vi "7. 绘制：管道内的 数据点分布 图.vi"(0 ">1000 数据点 红色":u32(colorbox)=13107200, 3 "<120 数据点 灰色":u32(colorbox)=11121611, 4 "<1000 数据点 橘色":u32(colorbox)=16732970, 5 "<-120 数据点 青色":u32(colorbox)=2817023, 6 "<400 数据点 黄色":u32(colorbox)=16769858, 7 "<-300 数据点 蓝色":u32(colorbox)=16777224, 8 "管道分布":picture, 9 "输入：放大倍数":i32, 10 "光纤分布":dbl[][](array[numeric]), 11 "数据分布 一维数组":dbl[](array[numeric]) format="%#_13g") -> (2 "管道+数据分布":picture)   [LabVIEW 2018]
panel:
  in  "fill?(F)":bool caption="填充？(F)"
  in  ">1000 数据点 画笔":T1={"Width"=8, "Style"=enum."Solid"}
  in  "<1000 数据点 画笔":T1={"Width"=8, "Style"=enum."Solid"}
  in  "<400 数据点 画笔":T1={"Width"=8, "Style"=enum."Solid"}
  in  ">1000 数据点：光纤+数据 分布":cluster{"x":dbl, "y":dbl, "数据":dbl, "索引":i32}[](array[cluster])
  in  "<1000 数据点：光纤+数据 分布":cluster{"x":dbl, "y":dbl, "数据":dbl, "索引":i32}[](array[cluster])
  in  "<400 数据点：光纤+数据 分布":cluster{"x":dbl, "y":dbl, "数据":dbl, "索引":i32}[](array[cluster])
  in  "<120 数据点 画笔":T1={"Width"=8, "Style"=enum."Solid"}
  in  "<-120 数据点 画笔":T1={"Width"=8, "Style"=enum."Solid"}
  in  "<120 数据点：光纤+数据 分布":cluster{"x":dbl, "y":dbl, "数据":dbl, "索引":i32}[](array[cluster])
  in  "<-120 数据点：光纤+数据 分布":cluster{"x":dbl, "y":dbl, "数据":dbl, "索引":i32}[](array[cluster])
  in  "<-300 数据点：光纤+数据 分布":cluster{"x":dbl, "y":dbl, "数据":dbl, "索引":i32}[](array[cluster])
  in  "<-300 数据点 画笔":T1={"Width"=8, "Style"=enum."Solid"}
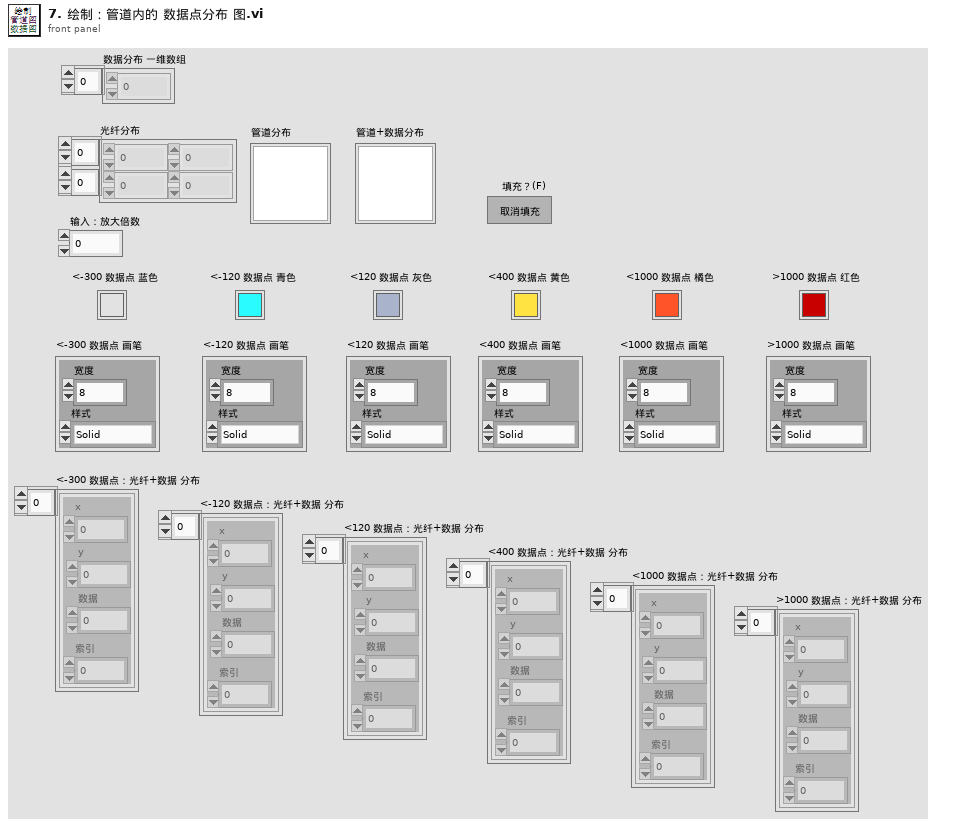
[diagram p1: front panel]
types:
  T1 = cluster{"Width":u16, "Style":enum32{"Solid", "Dash", "Dot", "DashDot", "DashDotDot"}}
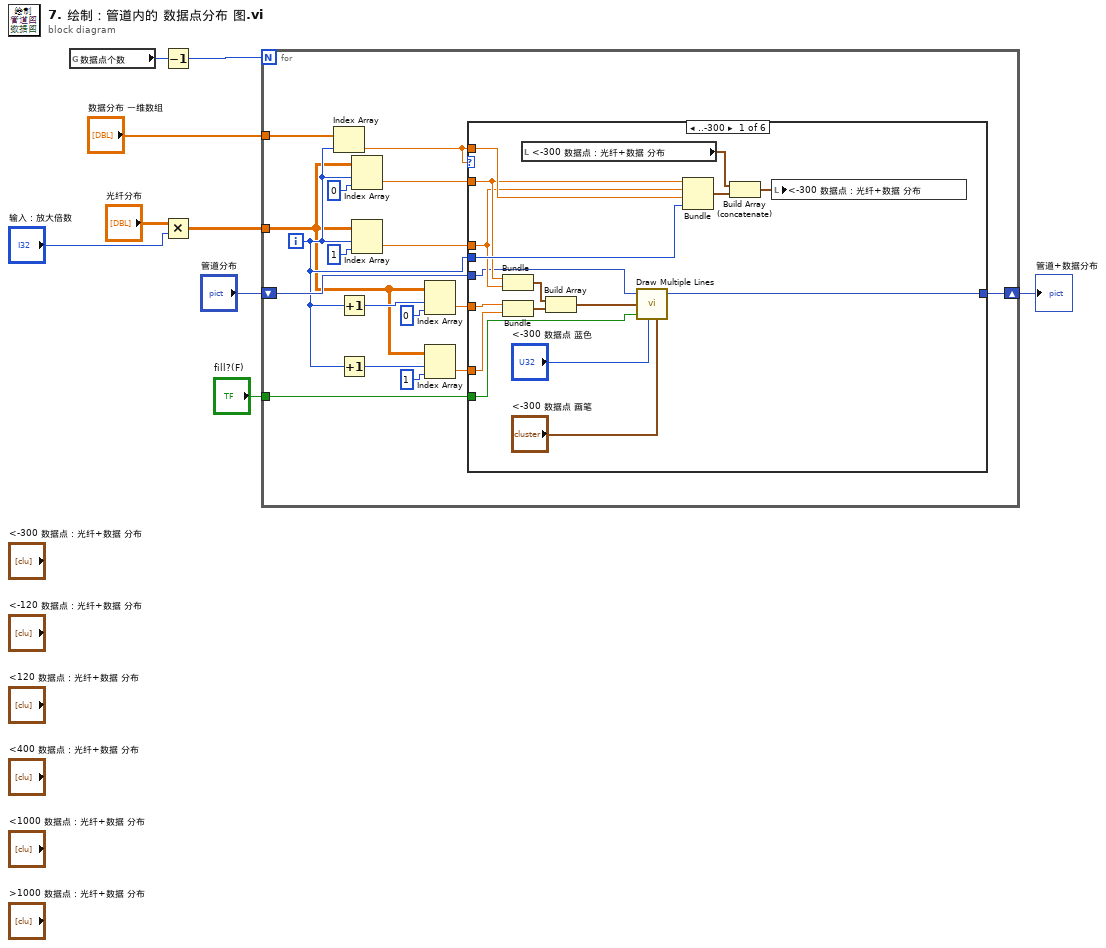
[diagram p0: block diagram]
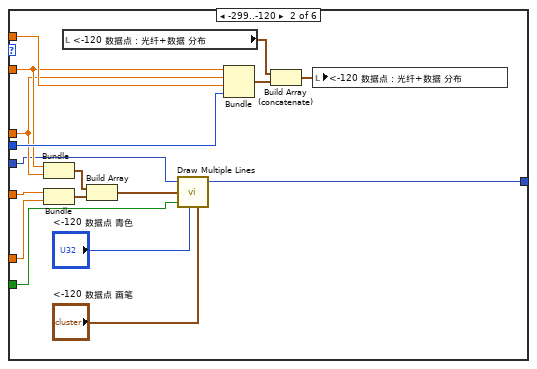
[diagram p2: hidden frame]
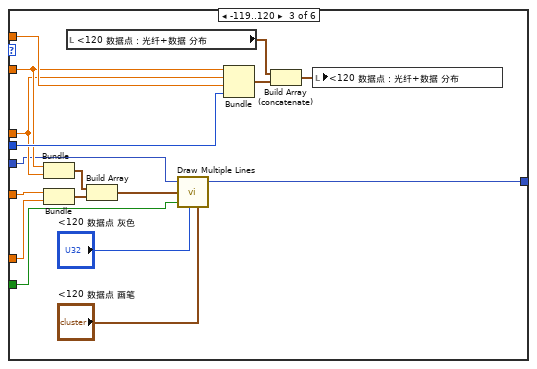
[diagram p3: hidden frame]
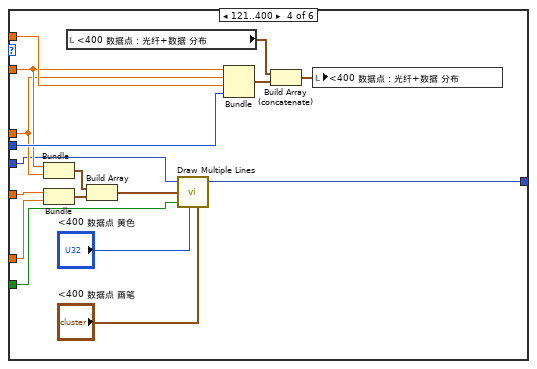
[diagram p4: hidden frame]
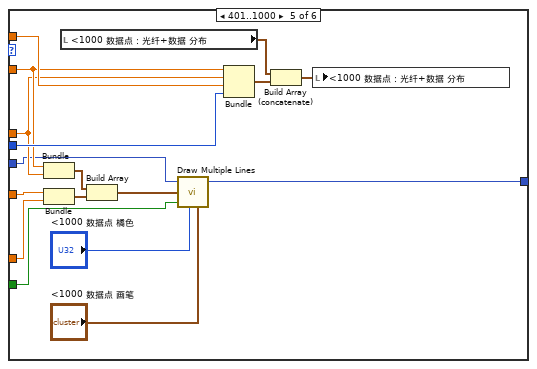
[diagram p5: hidden frame]
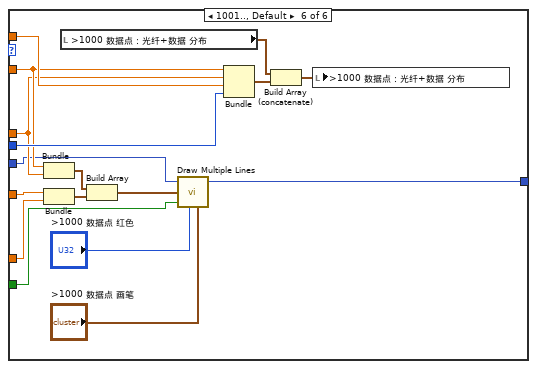
[diagram p6: hidden frame]
diagram:
  n1 = global read "全局变量：数据点个数.vi" "数据点个数"() -> (w2:i32)
  n2 = Decrement(x=w2) -> (x-1=w1:i32)
  n3 = Multiply(x="光纤分布", y="输入：放大倍数") -> (x*y=w9:dbl[][])
  n4 = for {
    N: w1 -> [_]
    tunnel: "数据分布 一维数组" -> [w26]
    tunnel: w9 -> [w13]
    shift-right: [w23] -> w4
    shift-left: "管道分布" -> [w20]
    tunnel: "fill?(F)" -> [w10]
    i -> [w14]
    n5 = Index Array(array=w26, index=w14) -> (element=w19:dbl)
    n6 = Increment(x=w14) -> (x+1=w16:i32)
    n7 = Increment(x=w14) -> (x+1=w15:i32)
    n8 = Index Array(array=w13, index (row)=w14, index (col)=0) -> (element=w22:dbl)
    n9 = Index Array(array=w13, index (row)=w14, index (col)=1) -> (element=w21:dbl)
    n10 = Index Array(array=w13, index (row)=w16, index (col)=0) -> (element=w12:dbl)
    n11 = Index Array(array=w13, index (row)=w15, index (col)=1) -> (element=w11:dbl)
    n12 = case shown="..-300" w19 {
      tunnel: w14 -> [w43 w60 w77 w94 w111 w128]
      tunnel: w19 -> [w42 w59 w76 w93 w110 w127]
      tunnel: w22 -> [w41 w58 w75 w92 w109 w126]
      tunnel: w21 -> [w40 w57 w74 w91 w108 w125]
      tunnel: w20 -> [w29 w47 w64 w79 w95 w113]
      tunnel: [w28 w48 w65 w82 w99 w112] -> w23
      tunnel: w12 -> [w36 w53 w70 w87 w104 w121]
      tunnel: w11 -> [w35 w52 w69 w86 w103 w120]
      tunnel: w10 -> [w27 w44 w61 w78 w98 w119]
      frame ..-300 {
        n13 = Bundle(w41, w40) -> (w33:cluster{dbl, dbl})  [unwired: 1 in]
        n14 = Bundle(w36, w35) -> (w34:cluster{dbl, dbl})  [unwired: 1 in]
        n15 = local read "<-300 数据点：光纤+数据 分布"() -> (w37:cluster{"x":dbl, "y":dbl, "数据":dbl, "索引":i32}[])
        n16 = Build Array(w33, w34) -> (w32:cluster{dbl, dbl}[])
        n17 = call <vilib>:"Draw Multiple Lines.vi"("picture"=w29, "line endpoints"=w32, "fill?(F)"=w27, "color(black)"="<-300 数据点 蓝色", "pen"="<-300 数据点 画笔") -> ("new picture"=w28:picture)  [unwired: 4 in]
        n18 = Bundle(w41, w40, "数值"=w42, w43) -> (w39:cluster{dbl, dbl, "数值":dbl, i32})  [unwired: 1 in]
        n19 = Build Array (concatenate)(w37, w39) -> (w38:cluster{"x":dbl, "y":dbl, "数值":dbl, "索引":i32}[])
        n20 = local write "<-300 数据点：光纤+数据 分布"(w38) -> ()
      }
      frame -299..-120 {
        n21 = Bundle(w58, w57) -> (w50:cluster{dbl, dbl})  [unwired: 1 in]
        n22 = Bundle(w53, w52) -> (w51:cluster{dbl, dbl})  [unwired: 1 in]
        n23 = local read "<-120 数据点：光纤+数据 分布"() -> (w54:cluster{"x":dbl, "y":dbl, "数据":dbl, "索引":i32}[])
        n24 = Build Array(w50, w51) -> (w49:cluster{dbl, dbl}[])
        n25 = call <vilib>:"Draw Multiple Lines.vi"("picture"=w47, "line endpoints"=w49, "fill?(F)"=w44, "color(black)"="<-120 数据点 青色", "pen"="<-120 数据点 画笔") -> ("new picture"=w48:picture)  [unwired: 4 in]
        n26 = Bundle(w58, w57, "数值"=w59, w60) -> (w56:cluster{dbl, dbl, "数值":dbl, i32})  [unwired: 1 in]
        n27 = Build Array (concatenate)(w54, w56) -> (w55:cluster{"x":dbl, "y":dbl, "数值":dbl, "索引":i32}[])
        n28 = local write "<-120 数据点：光纤+数据 分布"(w55) -> ()
      }
      frame -119..120 {
        n29 = Bundle(w75, w74) -> (w67:cluster{dbl, dbl})  [unwired: 1 in]
        n30 = Bundle(w70, w69) -> (w68:cluster{dbl, dbl})  [unwired: 1 in]
        n31 = local read "<120 数据点：光纤+数据 分布"() -> (w71:cluster{"x":dbl, "y":dbl, "数据":dbl, "索引":i32}[])
        n32 = Build Array(w67, w68) -> (w66:cluster{dbl, dbl}[])
        n33 = call <vilib>:"Draw Multiple Lines.vi"("picture"=w64, "line endpoints"=w66, "fill?(F)"=w61, "color(black)"="<120 数据点 灰色", "pen"="<120 数据点 画笔") -> ("new picture"=w65:picture)  [unwired: 4 in]
        n34 = Bundle(w75, w74, "数值"=w76, w77) -> (w73:cluster{dbl, dbl, "数值":dbl, i32})  [unwired: 1 in]
        n35 = Build Array (concatenate)(w71, w73) -> (w72:cluster{"x":dbl, "y":dbl, "数值":dbl, "索引":i32}[])
        n36 = local write "<120 数据点：光纤+数据 分布"(w72) -> ()
      }
      frame 121..400 {
        n37 = Bundle(w92, w91) -> (w84:cluster{dbl, dbl})  [unwired: 1 in]
        n38 = Bundle(w87, w86) -> (w85:cluster{dbl, dbl})  [unwired: 1 in]
        n39 = local read "<400 数据点：光纤+数据 分布"() -> (w88:cluster{"x":dbl, "y":dbl, "数据":dbl, "索引":i32}[])
        n40 = Build Array(w84, w85) -> (w83:cluster{dbl, dbl}[])
        n41 = call <vilib>:"Draw Multiple Lines.vi"("picture"=w79, "line endpoints"=w83, "fill?(F)"=w78, "color(black)"="<400 数据点 黄色", "pen"="<400 数据点 画笔") -> ("new picture"=w82:picture)  [unwired: 4 in]
        n42 = Bundle(w92, w91, "数值"=w93, w94) -> (w90:cluster{dbl, dbl, "数值":dbl, i32})  [unwired: 1 in]
        n43 = Build Array (concatenate)(w88, w90) -> (w89:cluster{"x":dbl, "y":dbl, "数值":dbl, "索引":i32}[])
        n44 = local write "<400 数据点：光纤+数据 分布"(w89) -> ()
      }
      frame 401..1000 {
        n45 = Bundle(w109, w108) -> (w101:cluster{dbl, dbl})  [unwired: 1 in]
        n46 = Bundle(w104, w103) -> (w102:cluster{dbl, dbl})  [unwired: 1 in]
        n47 = local read "<1000 数据点：光纤+数据 分布"() -> (w105:cluster{"x":dbl, "y":dbl, "数据":dbl, "索引":i32}[])
        n48 = Build Array(w101, w102) -> (w100:cluster{dbl, dbl}[])
        n49 = call <vilib>:"Draw Multiple Lines.vi"("picture"=w95, "line endpoints"=w100, "fill?(F)"=w98, "color(black)"="<1000 数据点 橘色", "pen"="<1000 数据点 画笔") -> ("new picture"=w99:picture)  [unwired: 4 in]
        n50 = Bundle(w109, w108, "数值"=w110, w111) -> (w107:cluster{dbl, dbl, "数值":dbl, i32})  [unwired: 1 in]
        n51 = Build Array (concatenate)(w105, w107) -> (w106:cluster{"x":dbl, "y":dbl, "数值":dbl, "索引":i32}[])
        n52 = local write "<1000 数据点：光纤+数据 分布"(w106) -> ()
      }
      frame 1001.., Default {
        n53 = Bundle(w126, w125) -> (w117:cluster{dbl, dbl})  [unwired: 1 in]
        n54 = Bundle(w121, w120) -> (w118:cluster{dbl, dbl})  [unwired: 1 in]
        n55 = local read ">1000 数据点：光纤+数据 分布"() -> (w122:cluster{"x":dbl, "y":dbl, "数据":dbl, "索引":i32}[])
        n56 = Build Array(w117, w118) -> (w116:cluster{dbl, dbl}[])
        n57 = call <vilib>:"Draw Multiple Lines.vi"("picture"=w113, "line endpoints"=w116, "fill?(F)"=w119, "color(black)"=">1000 数据点 红色", "pen"=">1000 数据点 画笔") -> ("new picture"=w112:picture)  [unwired: 4 in]
        n58 = Bundle(w126, w125, "数值"=w127, w128) -> (w124:cluster{dbl, dbl, "数值":dbl, i32})  [unwired: 1 in]
        n59 = Build Array (concatenate)(w122, w124) -> (w123:cluster{"x":dbl, "y":dbl, "数值":dbl, "索引":i32}[])
        n60 = local write ">1000 数据点：光纤+数据 分布"(w123) -> ()
      }
    }
  }
  "管道+数据分布" <- w4
